vi "Clock Cross Consumer Process.vi"(0 "read completion":T2, 2 "resources":T3, 12 "ready for output":bool) -> (4 "register instruction":T1)   [LabVIEW 2016]
doc: "Analogous to the register bus process VI. This VI outputs register instructions received from the other clock domain, returns read completions, and sends the ready for input signal from its attached registers to the other clock domain.\n\n<B>Input Parameters</B>\n\n<B>resources</B> contains references to the clock crossing FIFOs.\n\n<B>read completion</B> the output of the last executed register instruction.\n\n<B>ready for input</B> a flow control signal indicating whether the attached registers are ready for a new instruction. It is both sent to the other clock domain as well as used to halt instruction output from this VI.\n\n<B>Output Parameters</B>\n\n<B>register instruction</B> the register bus instruction to execute, sent from the other clock domain."
uses:
  Clock Cross Resources.ctl
  <instrlib>/_niInstr/Register Bus/v1/FPGA/Public/Read Completion.ctl
  <instrlib>/_niInstr/Register Bus/v1/FPGA/Public/Register Instruction.ctl
  <vilib>/rvi/DataTransferAndStorage/Container/Common/niFpgaContainerExecOnDevCompGetState.vi
  <vilib>/rvi/Emulation/niFpgaEmulationIsFPGAContextNoSignature.vi
  <vilib>/rvi/Emulation/niFpgaSctlEmulationGetInTimedLoop.vi
  <vilib>/rvi/errors/niFpgaSetErrorForExecOnDevCompSimple.vi
  <vilib>/rvi/eio/common/nirviEmuReportErrorAndStop.vi
  <vilib>/rvi/DataTransferAndStorage/Container/Common/niFpgaContainerGetUniqueNameForEmu.vi
  <vilib>/rvi/FIFO/Fifo_Resource/nirvififoEmulationSetSize.vi
  <vilib>/rvi/FIFO/Fifo_Resource/nirviFifoEmulationQueueMgr.vi
  <instcachedir>/0/nirviFifoEmulationQueueMgr_E5CAEC123FF24DC58D834DCA3CDAA9B5.lvgen/nirviFifoEmulationQueueMgr_E5CAEC123FF24DC58D834DCA3CDAA9B5_012.vi
  <vilib>/rvi/FIFO/Fifo_Resource/nirvififoEmulationDetermineInputValidOut.vi
  <vilib>/rvi/FIFO/Fifo_Resource/nirvififoEmulationCreateLock.vi
  <vilib>/rvi/Emulation/niFpgaProcessEmulError.vi
  <vilib>/rvi/FIFO/Fifo_Resource/nirvififoEmulationObtainLock.vi
  <vilib>/rvi/FIFO/Fifo_Resource/nirvififoEmulationReleaseLock.vi
  <vilib>/rvi/occurrence/nirviWaitOnOccurrenceBase.vi
  <vilib>/rvi/errors/nirviReportUnexpectedCaseInternalError.vi
  <vilib>/rvi/errors/nirviReportUnexpectedCaseInternalError (U32).vi
  <vilib>/Utility/error.llb/Clear Errors.vi
  <vilib>/rvi/interface/RandomDataEmulation/niFpgaRandomDataHandleErrors.vi
  <vilib>/rvi/DataTransferAndStorage/Container/XNode/niFpgaContainer.xnode
  <vilib>/rvi/FIFO/Fifo_Resource/niFpgaFifoEmulationRefIn.vi
  <vilib>/rvi/DataTransferAndStorage/Handshake/Emulation/niFpgaHandshakeEmulationRefIn.vi
  <instrlib>/_niInstr/Register Bus/v1/FPGA/niInstr Register Bus v1 FPGA.lvlib
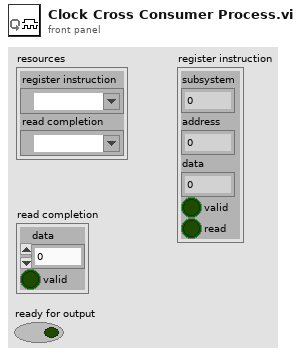
[diagram p1: front panel]
types:
  T1 = typedef "niInstr Register Bus v1 FPGA.lvlib/Register Instruction.ctl" = cluster{"subsystem":u8, "address":u16, "data":u32, "valid":bool, "read":bool}
  T2 = typedef "niInstr Register Bus v1 FPGA.lvlib/Read Completion.ctl" = cluster{"data":u32, "valid":bool}
  T3 = typedef "Clock Cross Resources.ctl" = cluster{"register instruction":refnum<k21>, "read completion":refnum<k21>}
  T4 = cluster{"subsystem":u8, "address":u16, "data":u32, "valid":bool, "read":bool}
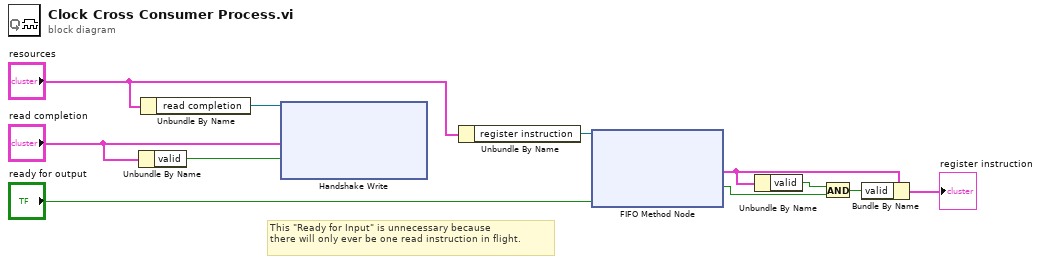
[diagram p0: block diagram]
diagram:
  # "This \"Ready for Input\" is unnecessary because\nthere will only ever be one read instruction in flight."
  n1 = Unbundle By Name("read completion") -> ("valid"=w2:bool)
  n2 = Unbundle By Name("resources") -> ("read completion"=w3:refnum<k21>)
  n3 = xnode "Handshake Write"("Data"="read completion", "Input Valid"=w2, "Handshake In"=w3) -> ()  [unwired: 2 out]
  n4 = Unbundle By Name("resources") -> ("register instruction"=w11:refnum<k21>)
  n5 = xnode ("FIFO Method Node")("Ready for Output"="ready for output", "FIFO In"=w11) -> ("Element"=w10:T4, "Output Valid"=w6:bool)  [unwired: 1 out]
  n6 = Unbundle By Name(w10) -> ("valid"=w7:bool)
  n7 = And(x=w7, y=w6) -> (x .and. y?=w5:bool)
  n8 = Bundle By Name(cluster=w10, "valid"=w5) -> (→"register instruction":T4)
